vi "Msg.vi"(7 "Actor in":refnum<class "Actor.lvclass">, 11 "Actor Destroy Msg Strategy in":refnum<class "Actor Destroy Msg Strategy.lvclass">) -> (0 "error out":errorcluster, 5 "Actor out":refnum<class "Actor.lvclass">)   [LabVIEW 2021, in "Actor Destroy.lvlib" / "Actor Destroy Msg Strategy.lvclass"]
uses:
  Actor Destroy Msg Strategy.lvclass
  LVCAM/Actor/Actor.lvclass
  Actor Destroy/Actor Destroy.lvclass
  8b074ebc-55b2-44bc-a317-0de79f881938.vi
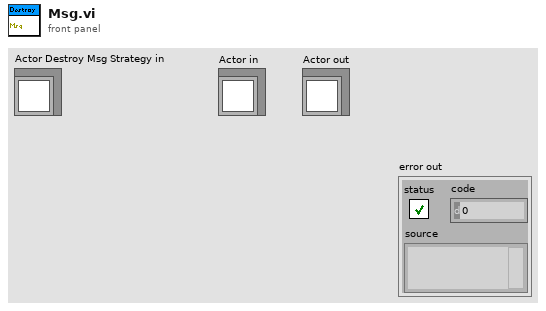
[diagram p1: front panel]
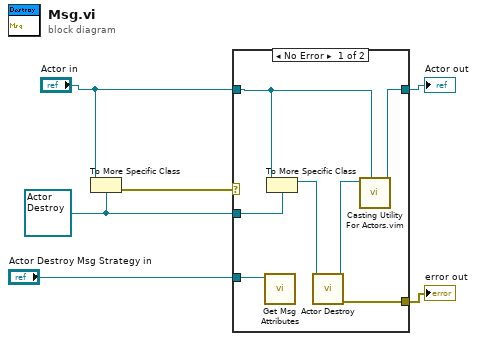
[diagram p0: block diagram]
diagram:
  w2 = refnum<class "Actor Destroy.lvclass"> refnum ("Destroy.lvlib:Destroy.lvclass")
  n1 = To More Specific Class(target class=w2, reference="Actor in") -> (error out=w6:errorcluster)  [unwired: 1 in, 1 out]
  n2 = case shown="No Error" w6 {
    selector: w6 -> [_ w15]
    tunnel: [w7 w15] -> w1
    tunnel: [w12 w14] -> w3
    tunnel: "Actor in" -> [w11 w14]
    tunnel: w2 -> [w13 _]
    tunnel: "Actor Destroy Msg Strategy in" -> [w10 _]
    frame No Error {
      n3 = call "Get Msg Attributes.vi"("Actor Destroy Msg Strategy in"=w10) -> ()  [unwired: 11 in]
      n4 = To More Specific Class(target class=w13, reference=w11) -> (specific class reference=w9:refnum<class "Actor Destroy.lvclass">)  [unwired: 1 in, 1 out]
      n5 = call-dynamic "Actor Destroy.vi"("Actor Destroy in"=w9) -> ("error out"=w7:errorcluster, "Actor Destroy out"=w8:refnum<class "Actor Destroy.lvclass">)  [unwired: 9 in]
      n6 = call "Casting Utility For Actors.vim"("type"=w11, "Actor in"=w8) -> ("Actor out"=w12:refnum<class "Actor.lvclass">)  [unwired: 8 in, 1 out]
    }
    frame Error {
    }
  }
  "error out" <- w1
  "Actor out" <- w3
